vi "Set Power.vi"(8 "error in (no error)":errorcluster, 10 "Power":dbl, 11 "Laser Process in":refnum<class "Laser Process.lvclass">) -> (0 "error out":errorcluster, 3 "Laser Process out":refnum<class "Laser Process.lvclass">)   [LabVIEW 2022 SP3, in "Laser Process.lvlib" / "Laser Process.lvclass"]
uses:
  Laser Process.lvclass
  Laser Process.lvclass/Laser Process.ctl
  Laser Driver/Laser Driver.lvclass
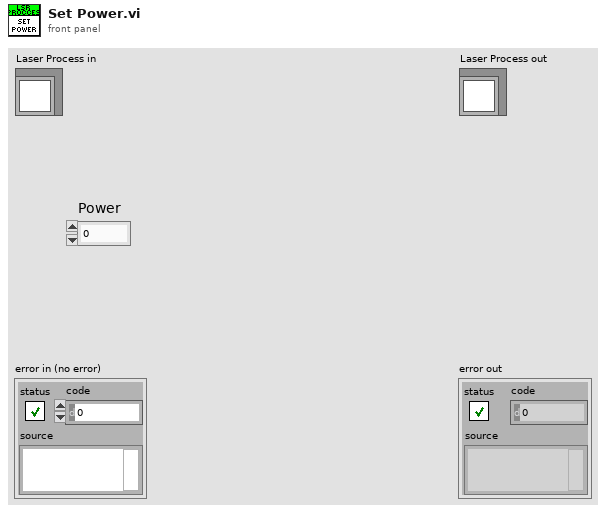
[diagram p1: front panel]
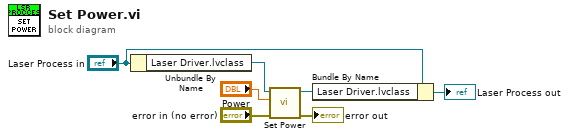
[diagram p0: block diagram]
diagram:
  n1 = Unbundle By Name("Laser Process in") -> ("Laser Driver.lvclass"=w6:refnum<class "Laser Driver.lvclass">)
  n2 = call-dynamic "Set Power.vi"("error in (no error)"="error in (no error)", "Power Percentage"="Power", "Laser Driver in"=w6) -> ("error out"=→"error out":errorcluster, "Laser Driver out"=w1:refnum<class "Laser Driver.lvclass">)  [unwired: 7 in]
  n3 = Bundle By Name(cluster="Laser Process in", "Laser Driver.lvclass"=w1) -> (→"Laser Process out":refnum<class "Laser Process.lvclass">)
